vi "Autonomous.vi"() -> ()   [LabVIEW 2018]
doc: "This VI starts when autonomous period begins, and will automatically be terminated when it ends. You can carry out timed or sensor driven operations directly to I/O or to subsystems without needing to return to the caller."
uses:
  Motion_Profiler_Class-master/MotionProfiles.lvclass
  <vilib>/Rock Robotics/WPI/SafetyOutput/WPI_SafetyOutputConfigMenu.ctl
  d1af4e31-2977-4334-b470-f567b7f2c4f2.vi
  <vilib>/Rock Robotics/Network Tables/NT Read String.vi
  <vilib>/Rock Robotics/WPI/Utilities/WPI_GetSetVariantRefNum.vi
  <vilib>/Rock Robotics/Network Tables/NT Read Boolean.vi
panel:
  out "MotionProfiles out":refnum<class "MotionProfiles.lvclass">
  out "Left Motor":T1(graph)
  out "Left Throttle":dbl(graph)
  out "Right Motor":T2(graph)
  out "Right Throttle":dbl(graph)
  out "Right Bottom Buf Count":i32
  out "Left Bottom Buf Count":i32
  out "Right Under Run":bool
  out "Left Under Run":bool
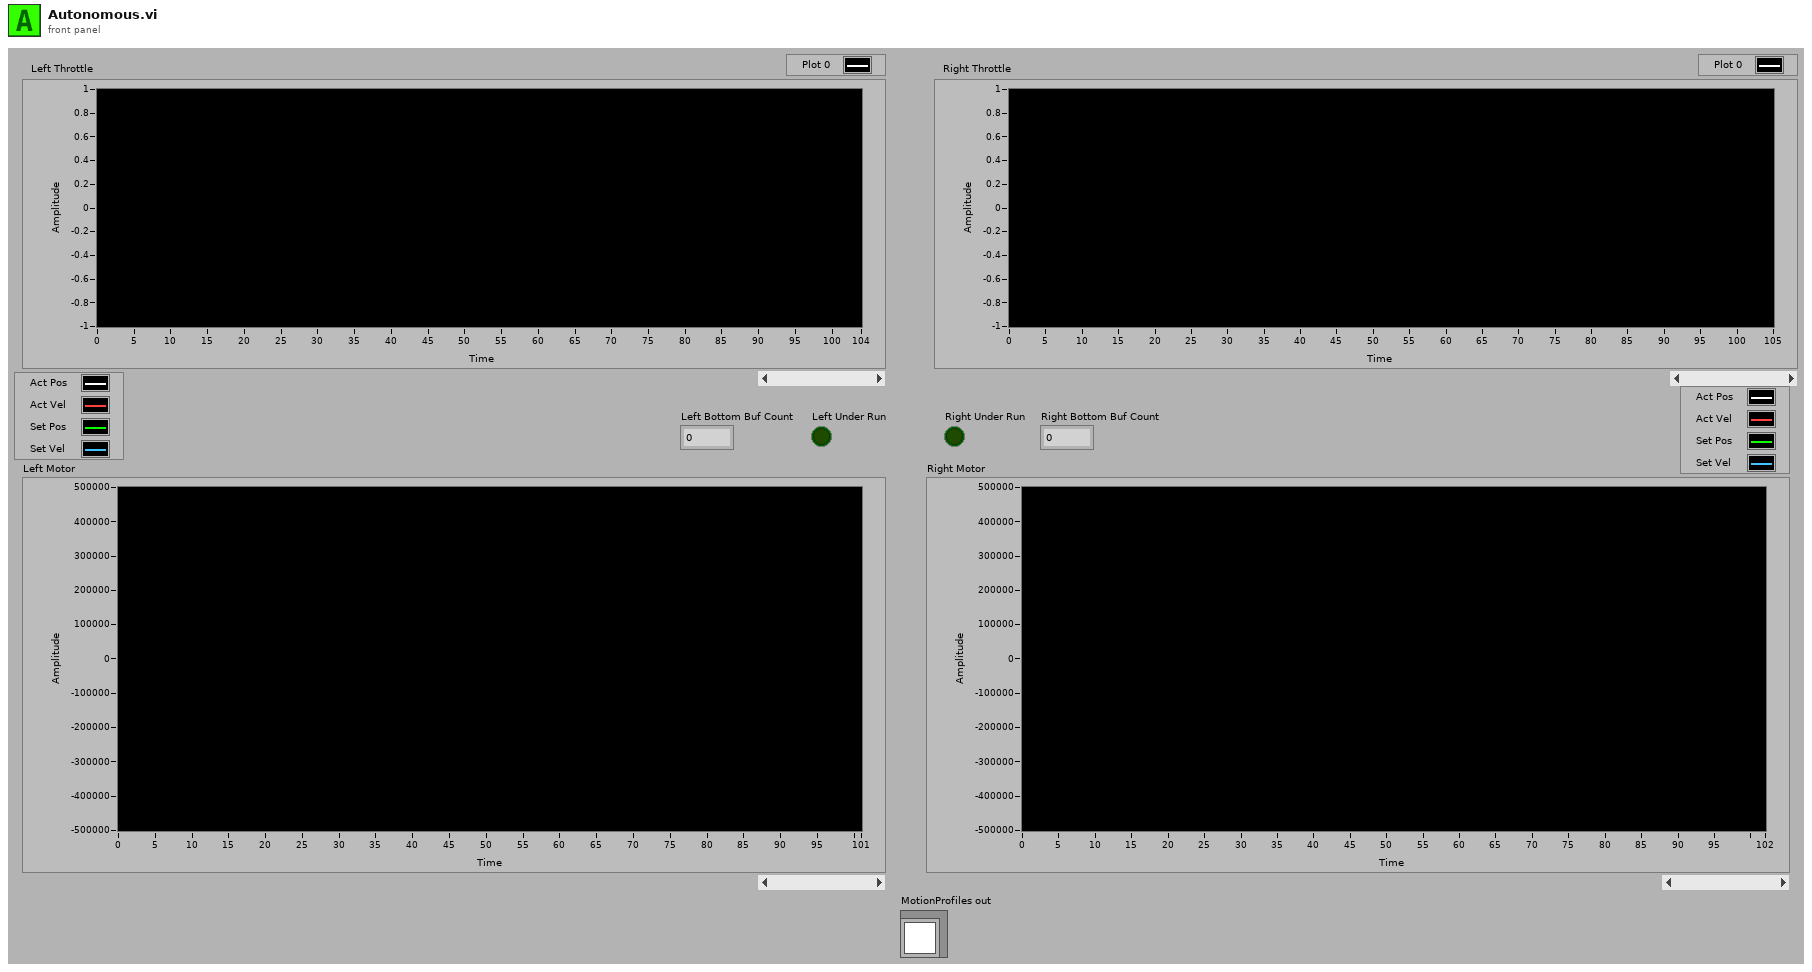
[diagram p1: front panel]
types:
  T1 = cluster{"Set_Pos_(u)":i32, "Set_Pos_(u)":i32, "Act_Vel_(u/100ms)":i32, "Set_Vel_(u/100ms)":i32}
  T2 = cluster{"Set_Vel_(u/100ms)":i32, "Act_Vel_(u/100ms)":i32, "Set_Pos_(u)":i32, "Act_Pos(u)":i32}
  T3 = typedef "WPI_SafetyOutputConfigMenu.ctl" = enum16{"Enable", "Disable"}
  T4 = typedef "WPI_RobotDriveDevRef.ctl" = cluster{"DevStatus":errorcluster, "Motors[]":T5[], "Square Inputs":bool, "Max Output":dbl}
  T5 = typedef "WPI_MotorControlDeviceRef.ctl" = cluster{"DeviceStatus":errorcluster, "Type":T6, "PWM":cluster{"PWM Channel":T7, "DeadBand":T8}, "CAN":cluster{"Device Number":u8, "SetOutput VI Ref":variant, "GetOutput VI Ref":variant, "Enable VI Ref":variant, "Disable VI Ref":variant, "Data":variant}, "Invert":bool, "DIO PWM":cluster{"PWM \"Enable\" Channel":T7, "DIOChannel":T9, "PWM Rate":dbl}}
  T6 = typedef "WPI_MotorControlType.ctl" = enum16{"PWM", "CAN", "DIO PWM"}
  T7 = typedef "FPGA_DIOPWMChannel.ctl" = enum8{"PWM 0", "PWM 1", "PWM 2", "PWM 3", "PWM 4", "PWM 5", "PWM 6", "PWM 7", "PWM 8", "PWM 9", "PWM MXP 0", "PWM MXP 1", "PWM MXP 2", "PWM MXP 3", "PWM MXP 4", "PWM MXP 5", "PWM MXP 6", "PWM MXP 7", "PWM MXP 8", "PWM MXP 9", "Invalid"}
  T8 = typedef "WPI_PWMDeadband.ctl" = cluster{"Name":string, "maxPositivePwm":i32, "minPositivePwm":i32, "centerPwm":i32, "maxNegativePwm":i32, "minNegativePwm":i32, "angularRange":u16}
  T9 = typedef "FPGA_DIOChannel.ctl" = enum8{"DIO 0", "DIO 1", "DIO 2", "DIO 3", "DIO 4", "DIO 5", "DIO 6", "DIO 7", "DIO 8", "DIO 9", "DIO MXP 0", "DIO MXP 1", "DIO MXP 2", "DIO MXP 3", "DIO MXP 4", "DIO MXP 5", "DIO MXP 6", "DIO MXP 7", "DIO MXP 8", "DIO MXP 9", "DIO MXP 10", "DIO MXP 11", "DIO MXP 12", "DIO MXP 13", "DIO MXP 14", "DIO MXP 15", "SPI Port CS1", "SPI Port CS2", "SPI Port CS3", "SPI Port MISO", "SPI Port MOSI", "Invalid"}
  T10 = typedef "MotionProfiles.lvclass/MotionProfile_MP_Class_Status.ctl" = cluster{"Motion Profile Status":cluster{"Top Buffer Remaining":i32, "Top Buffer Count":i32, "Bottom Buffer Count":i32, "Has Underrun?":bool, "Is Underrun?":bool, "Active Point Valid?":bool, "Is Last?":bool, "Profile Slot Select 0":i32, "Output Enable":i32, "Time Duration (ms)":i32, "Profile Slot Select 1":i32}, "TalonState":T11, "MP Is Done":bool, "MP Is Executing":bool, "Set_Vel_(u/100ms)":i32, "Set_Pos_(u)":i32, "Act_Vel_(u/100ms)":i32, "Act_Pos(u)":i32, "Throtle":dbl}
  T11 = typedef "MotionProfiles.lvclass/MotionProfile_TalonSetValueEnum.ctl" = enum16{"Disable", "Enable", "Hold"}
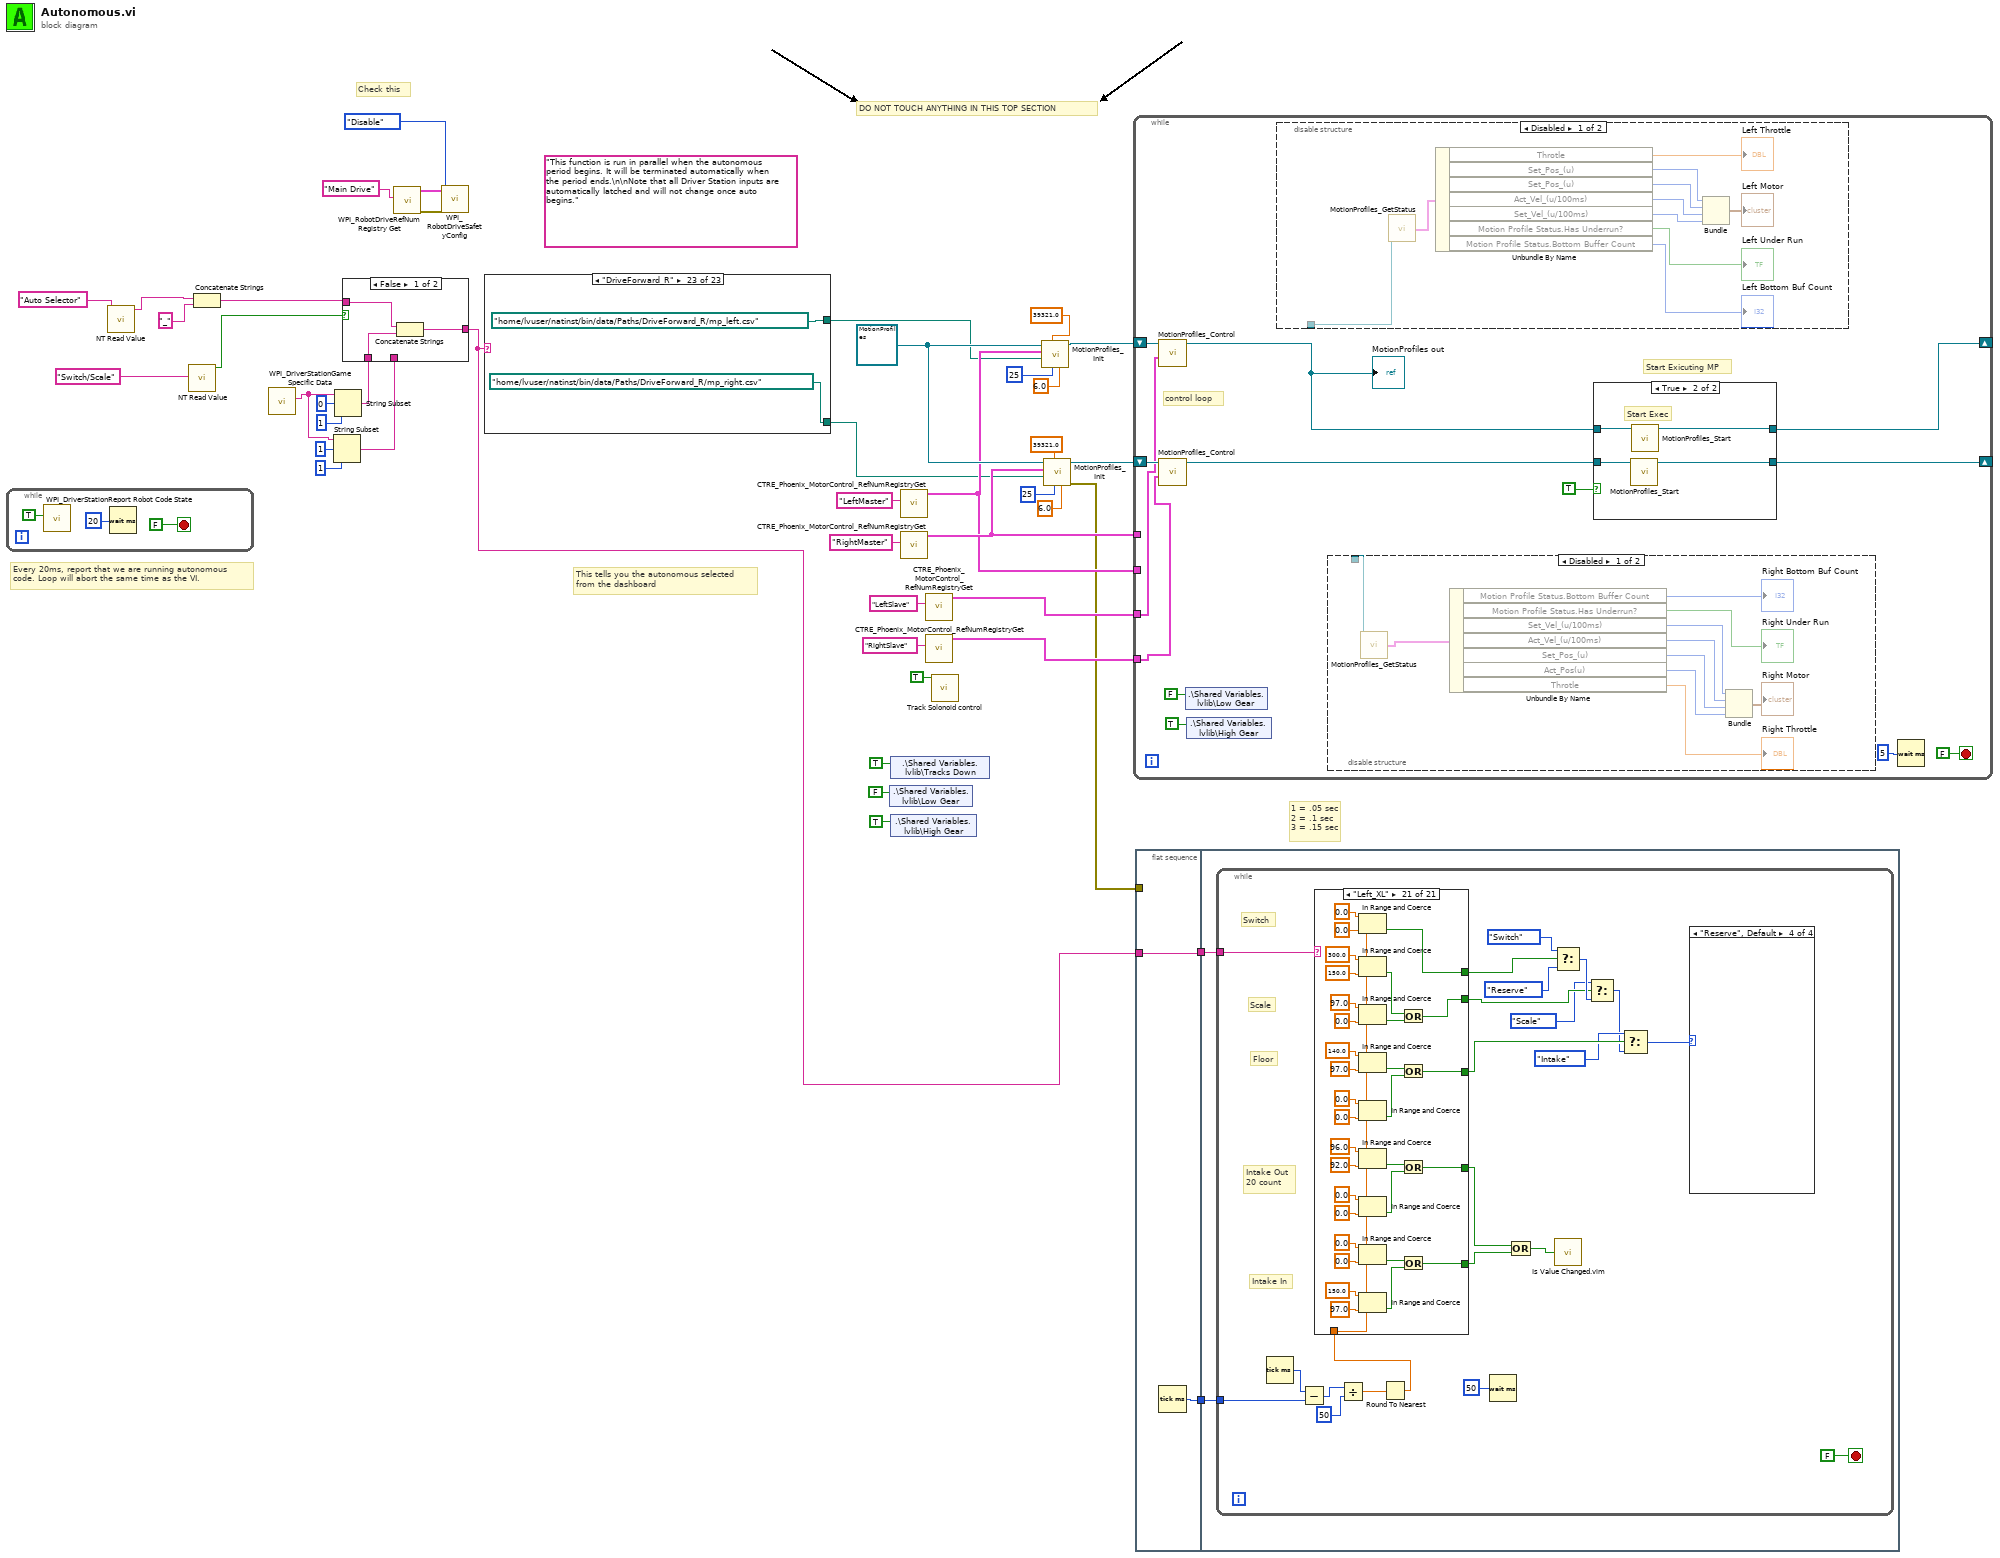
[diagram p0: block diagram]
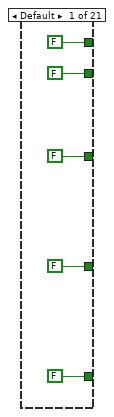
[diagram p5: hidden frame]
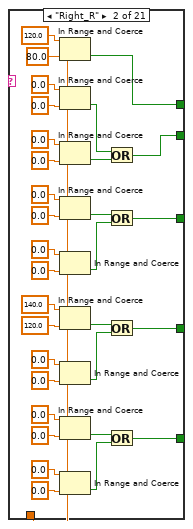
[diagram p6: hidden frame]
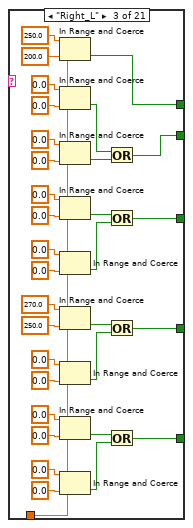
[diagram p7: hidden frame]
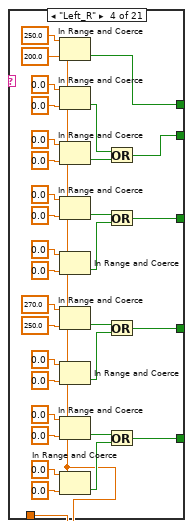
[diagram p8: hidden frame]
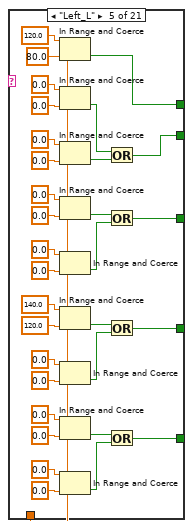
[diagram p9: hidden frame]
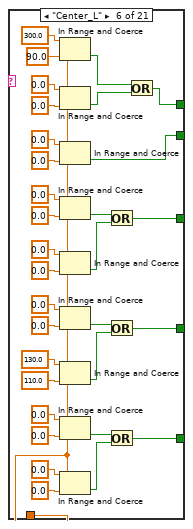
[diagram p10: hidden frame]
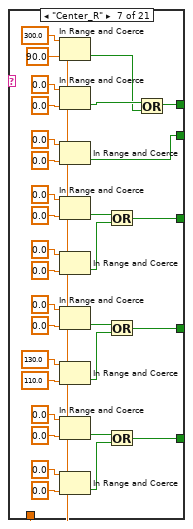
[diagram p11: hidden frame]
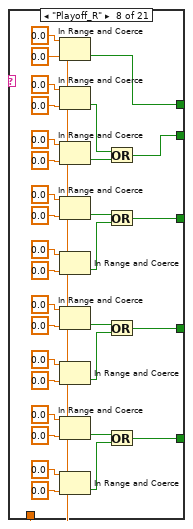
[diagram p12: hidden frame]
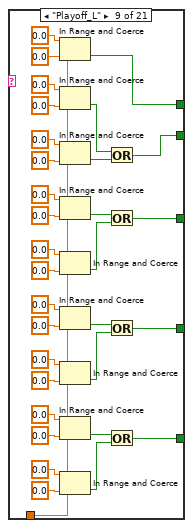
[diagram p13: hidden frame]
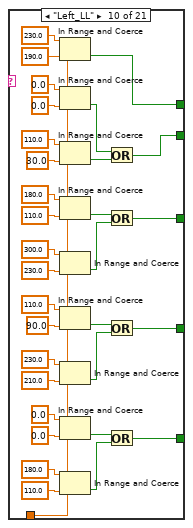
[diagram p14: hidden frame]
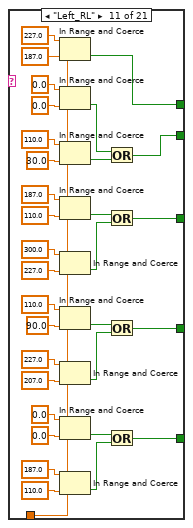
[diagram p15: hidden frame]
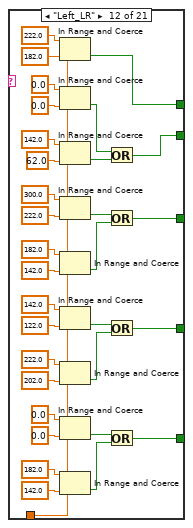
[diagram p16: hidden frame]
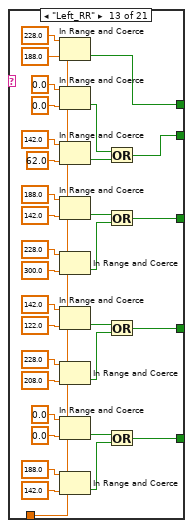
[diagram p17: hidden frame]
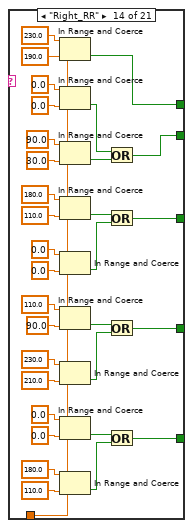
[diagram p18: hidden frame]
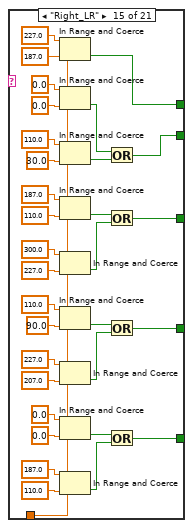
[diagram p19: hidden frame]
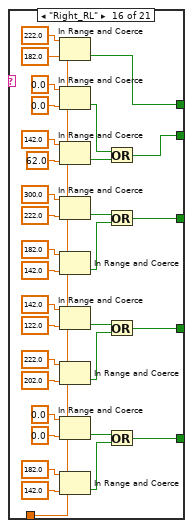
[diagram p20: hidden frame]
diagram:
  w40 = refnum<class "MotionProfiles.lvclass"> refnum ("MotionProfiles.lvclass")
  (unwired) "This function is run in parallel when the autonomous period begins. It will be terminated automatically when the period ends.\n\nNote that all Driver Station inputs are automatically latched and will not change once auto begins."
  # "1 = .05 sec\n2 = .1 sec\n3 = .15 sec"
  # "Check this"
  # "DO NOT TOUCH ANYTHING IN THIS TOP SECTION"
  # "This tells you the autonomous selected\nfrom the dashboard"
  # "Every 20ms, report that we are running autonomous\ncode. Loop will abort the same time as the VI."
  n1 = while {
    stop <- FALSE stop-if-true
    n2 = call <vilib>:"WPI_DriverStationReport Robot Code State.vi"("Autonomous"=TRUE) -> ()  [unwired: 10 in, 1 out]
    n3 = Wait (ms)(milliseconds to wait=u32 20) -> ()  [unwired: 1 out]
  }
  n4 = call-poly <vilib>:"NT Read Value.vi"("Name"="Auto Selector") -> ("String"=w18:string)  [unwired: 9 in, 1 out]
  n5 = call-poly <vilib>:"NT Read Value.vi"("Name"="Switch/Scale") -> ("Boolean"=w4:bool)  [unwired: 9 in, 1 out]
  n6 = Concatenate Strings(w18, "_" ("string")) -> (w8:string)
  n7 = call <vilib>:"WPI_DriverStationGame Specific Data.vi"() -> ("Game Specific Data"=w9:string)  [unwired: 11 in]
  n8 = String Subset(string=w9, offset (0)=1, length (rest)=1 ("length (rest)")) -> (substring=w7:string)
  n9 = String Subset(string=w9, offset (0)=0, length (rest)=1 ("length (rest)")) -> (substring=w6:string)
  n10 = case shown="False" w4 {
    tunnel: w8 -> [w49 w54]
    tunnel: w7 -> [_ w53]
    tunnel: w6 -> [w50 _]
    tunnel: [w48 w52] -> w5
    frame False {
      n11 = Concatenate Strings(w49, w50) -> (w48:string)
    }
    frame True {
      n12 = Concatenate Strings(w54, "X" ("string"), w53) -> (w52:string)
    }
  }
  n13 = call <vilib>:"WPI_RobotDriveRefNum Registry Get.vi"("refnum name"="Main Drive") -> ("error out"=w16:errorcluster, "RobotDriveDevRef"=w15:T4)  [unwired: 9 in]
  n14 = call <vilib>:"WPI_RobotDriveSafetyConfig.vi"("error in (no error)"=w16, "mode"=WPI_SafetyOutputConfigMenu."Disable", "RobotDriveDevRef"=w15) -> ()  [unwired: 7 in, 2 out]
  n15 = case shown="\"DriveForward_R\"" w5 {
    tunnel: [path "" path "/home/lvuser/natinst/bin/data/Paths/Left_L/mp_right.csv" ("file path (use dialog)") path "/home/lvuser/natinst/bin/data/Paths/Left_R/mp_right.csv" ("file path (use dialog)") path "/home/lvuser/natinst/bin/data/Paths/Center_R/mp_right.csv" ("file path (use dialog)") path "/home/lvuser/natinst/bin/data/Paths/Center_L/mp_right.csv" ("file path (use dialog)") path "/home/lvuser/natinst/bin/data/Paths/Right_L/mp_right.csv" ("file path (use dialog)") path "/home/lvuser/natinst/bin/data/Paths/Right_R/mp_right.csv" ("file path (use dialog)") path "/home/lvuser/natinst/bin/data/Paths/Playoff_R/mp_right.csv" ("file path (use dialog)") path "/home/lvuser/natinst/bin/data/Paths/Playoff_L/mp_right.csv" ("file path (use dialog)") path "/home/lvuser/natinst/bin/data/Paths/Left_LL/mp_right.csv" ("file path (use dialog)") path "/home/lvuser/natinst/bin/data/Paths/Left_RL/mp_right.csv" ("file path (use dialog)") path "/home/lvuser/natinst/bin/data/Paths/Left_LR/mp_right.csv" ("file path (use dialog)") path "/home/lvuser/natinst/bin/data/Paths/Left_RR/mp_right.csv" ("file path (use dialog)") path "/home/lvuser/natinst/bin/data/Paths/Right_LL/mp_right.csv" ("file path (use dialog)") path "/home/lvuser/natinst/bin/data/Paths/Right_LR/mp_right.csv" ("file path (use dialog)") path "/home/lvuser/natinst/bin/data/Paths/Right_RL/mp_right.csv" ("file path (use dialog)") path "/home/lvuser/natinst/bin/data/Paths/Right_RR/mp_right.csv" ("file path (use dialog)") path "/home/lvuser/natinst/bin/data/Paths/Left_XL/mp_right.csv" ("file path (use dialog)") path "/home/lvuser/natinst/bin/data/Paths/Left_XR/mp_right.csv" ("file path (use dialog)") path "/home/lvuser/natinst/bin/data/Paths/Right_XR/mp_right.csv" ("file path (use dialog)") path "/home/lvuser/natinst/bin/data/Paths/Right_XL/mp_right.csv" ("file path (use dialog)") path "/home/lvuser/natinst/bin/data/Paths/DriveForward_L/mp_right.csv" ("file path (use dialog)") path "/home/lvuser/natinst/bin/data/Paths/DriveForward_R/mp_right.csv" ("file path (use dialog)")] -> w13
    tunnel: [path "" path "/home/lvuser/natinst/bin/data/Paths/Left_L/mp_left.csv" ("file path (use dialog)") path "/home/lvuser/natinst/bin/data/Paths/Left_R/mp_left.csv" ("file path (use dialog)") path "/home/lvuser/natinst/bin/data/Paths/Center_R/mp_left.csv" ("file path (use dialog)") path "/home/lvuser/natinst/bin/data/Paths/Center_L/mp_left.csv" ("file path (use dialog)") path "/home/lvuser/natinst/bin/data/Paths/Right_L/mp_left.csv" ("file path (use dialog)") path "/home/lvuser/natinst/bin/data/Paths/Right_R/mp_left.csv" ("file path (use dialog)") path "/home/lvuser/natinst/bin/data/Paths/Playoff_R/mp_left.csv" ("file path (use dialog)") path "/home/lvuser/natinst/bin/data/Paths/Playoff_L/mp_left.csv" ("file path (use dialog)") path "/home/lvuser/natinst/bin/data/Paths/Left_LL/mp_left.csv" ("file path (use dialog)") path "/home/lvuser/natinst/bin/data/Paths/Left_RL/mp_left.csv" ("file path (use dialog)") path "/home/lvuser/natinst/bin/data/Paths/Left_LR/mp_left.csv" ("file path (use dialog)") path "/home/lvuser/natinst/bin/data/Paths/Left_RR/mp_left.csv" ("file path (use dialog)") path "/home/lvuser/natinst/bin/data/Paths/Right_LL/mp_left.csv" ("file path (use dialog)") path "/home/lvuser/natinst/bin/data/Paths/Right_LR/mp_left.csv" ("file path (use dialog)") path "/home/lvuser/natinst/bin/data/Paths/Right_RL/mp_left.csv" ("file path (use dialog)") path "/home/lvuser/natinst/bin/data/Paths/Right_RR/mp_left.csv" ("file path (use dialog)") path "/home/lvuser/natinst/bin/data/Paths/Left_XL/mp_left.csv" ("file path (use dialog)") path "/home/lvuser/natinst/bin/data/Paths/Left_XR/mp_left.csv" ("file path (use dialog)") path "/home/lvuser/natinst/bin/data/Paths/Right_XR/mp_left.csv" ("file path (use dialog)") path "/home/lvuser/natinst/bin/data/Paths/Right_XL/mp_left.csv" ("file path (use dialog)") path "/home/lvuser/natinst/bin/data/Paths/DriveForward_L/mp_left.csv" ("file path (use dialog)") path "/home/lvuser/natinst/bin/data/Paths/DriveForward_R/mp_left.csv" ("file path (use dialog)")] -> w12
    frame Default {
    }
    frame "Left_L" {
    }
    frame "Left_R" {
    }
    frame "Center_R" {
    }
    frame "Center_L" {
    }
    frame "Right_L" {
    }
    frame "Right_R" {
    }
    frame "Playoff_R" {
    }
    frame "Playoff_L" {
    }
    frame "Left_LL" {
    }
    frame "Left_RL" {
    }
    frame "Left_LR" {
    }
    frame "Left_RR" {
    }
    frame "Right_LL" {
    }
    frame "Right_LR" {
    }
    frame "Right_RL" {
    }
    frame "Right_RR" {
    }
    frame "Left_XL" {
    }
    frame "Left_XR" {
    }
    frame "Right_XR" {
    }
    frame "Right_XL" {
    }
    frame "DriveForward_L" {
    }
    frame "DriveForward_R" {
    }
  }
  n16 = shared-variable ".\\Shared Variables.lvlib\\Low Gear"(FALSE ("Low Gear")) -> ()  [unwired: 1 in, 1 out]
  n17 = shared-variable ".\\Shared Variables.lvlib\\Tracks Down"(TRUE ("High Gear")) -> ()  [unwired: 1 in, 1 out]
  n18 = shared-variable ".\\Shared Variables.lvlib\\High Gear"(TRUE ("High Gear")) -> ()  [unwired: 1 in, 1 out]
  n19 = call <vilib>:"CTRE_Phoenix_MotorControl_RefNumRegistryGet.vi"("refnum name"="LeftMaster") -> ("PhoenixMotorControlDevRef"=w31:T5)  [unwired: 9 in, 1 out]
  n20 = call <vilib>:"CTRE_Phoenix_MotorControl_RefNumRegistryGet.vi"("refnum name"="RightMaster") -> ("PhoenixMotorControlDevRef"=w32:T5)  [unwired: 9 in, 1 out]
  n21 = call <vilib>:"CTRE_Phoenix_MotorControl_RefNumRegistryGet.vi"("refnum name"="LeftSlave") -> ("PhoenixMotorControlDevRef"=w25:T5)  [unwired: 9 in, 1 out]
  n22 = call <vilib>:"CTRE_Phoenix_MotorControl_RefNumRegistryGet.vi"("refnum name"="RightSlave") -> ("PhoenixMotorControlDevRef"=w24:T5)  [unwired: 9 in, 1 out]
  n23 = call "Track Solonoid control.vi"("Manual Tracks"=TRUE) -> ()  [unwired: 11 in]
  n24 = call "MotionProfiles_Init.vi"("Wheel_Diameter (in)"=6.0 ("Wheel Diameter"), "MP_Frame_Rate_(ms)"=25, "Encoder_CPR_4x"=39321.0, "CSV File Path"=w12, "PhoenixMotorControlDevRef"=w31, "MotionProfiles in"=w40) -> ("MotionProfiles out"=w43:refnum<class "MotionProfiles.lvclass">)  [unwired: 4 in, 1 out]
  n25 = call "MotionProfiles_Init.vi"("Wheel_Diameter (in)"=6.0, "MP_Frame_Rate_(ms)"=25, "Encoder_CPR_4x"=39321.0, "CSV File Path"=w13, "PhoenixMotorControlDevRef"=w32, "MotionProfiles in"=w40) -> ("error out"=w23:errorcluster, "MotionProfiles out"=w41:refnum<class "MotionProfiles.lvclass">)  [unwired: 4 in]
  n26 = while {
    shift-right: [w108] -> _
    shift-left: w43 -> [w111]
    shift-right: [w109] -> _
    shift-left: w41 -> [w110]
    tunnel: w32 -> [_]
    tunnel: w31 -> [_]
    tunnel: w25 -> [w106]
    tunnel: w24 -> [w105]
    stop <- FALSE stop-if-true
    # "control loop"
    # "Start Exicuting MP"
    n27 = call "MotionProfiles_Control.vi"("PhoenixMotorControlDevRef Slave"=w106, "MotionProfiles in"=w111) -> ("MotionProfiles out"=w101:refnum<class "MotionProfiles.lvclass">)  [unwired: 8 in, 1 out]
    "MotionProfiles out" <- w101
    n28 = call "MotionProfiles_Control.vi"("PhoenixMotorControlDevRef Slave"=w105, "MotionProfiles in"=w110) -> ("MotionProfiles out"=w102:refnum<class "MotionProfiles.lvclass">)  [unwired: 8 in, 1 out]
    n29 = shared-variable ".\\Shared Variables.lvlib\\Low Gear"(FALSE ("Low Gear")) -> ()  [unwired: 1 in, 1 out]
    n30 = shared-variable ".\\Shared Variables.lvlib\\High Gear"(TRUE ("High Gear")) -> ()  [unwired: 1 in, 1 out]
    n31 = disable-structure shown="Disabled" {
      disable-tunnel: _ -> [w133 _]
      frame Disabled {
        n32 = call "MotionProfiles_GetStatus.vi"("MotionProfiles in"=w133) -> ("MP_Class_Status"=w132:T10)  [unwired: 12 in, 2 out]
        n33 = Unbundle By Name(w132) -> ("Throtle"=→"Left Throttle":dbl, "Set_Pos_(u)"=w125:i32, "Set_Pos_(u)"=w126:i32, "Act_Vel_(u/100ms)"=w127:i32, "Set_Vel_(u/100ms)"=w128:i32, "Motion Profile Status.Has Underrun?"=→"Left Under Run":bool, "Motion Profile Status.Bottom Buffer Count"=→"Left Bottom Buf Count":i32)
        n34 = Bundle("Set_Pos_(u)"=w125, "Set_Pos_(u)"=w126, "Act_Vel_(u/100ms)"=w127, "Set_Vel_(u/100ms)"=w128) -> (→"Left Motor":T1)  [unwired: 1 in]
      }
      frame Enabled {
      }
    }
    n35 = disable-structure shown="Disabled" {
      disable-tunnel: _ -> [w123 _]
      frame Disabled {
        n36 = call "MotionProfiles_GetStatus.vi"("MotionProfiles in"=w123) -> ("MP_Class_Status"=w122:T10)  [unwired: 12 in, 2 out]
        n37 = Unbundle By Name(w122) -> ("Motion Profile Status.Bottom Buffer Count"=→"Right Bottom Buf Count":i32, "Motion Profile Status.Has Underrun?"=→"Right Under Run":bool, "Set_Vel_(u/100ms)"=w118:i32, "Act_Vel_(u/100ms)"=w117:i32, "Set_Pos_(u)"=w116:i32, "Act_Pos(u)"=w115:i32, "Throtle"=→"Right Throttle":dbl)
        n38 = Bundle("Set_Vel_(u/100ms)"=w118, "Act_Vel_(u/100ms)"=w117, "Set_Pos_(u)"=w116, "Act_Pos(u)"=w115) -> (→"Right Motor":T2)  [unwired: 1 in]
      }
      frame Enabled {
      }
    }
    n39 = case shown="True" TRUE {
      tunnel: w101 -> [w135 w139]
      tunnel: w102 -> [w134 w137]
      tunnel: [w134 w136] -> w109
      tunnel: [w135 w138] -> w108
      frame False {
      }
      frame True {
        # "Start Exec"
        n40 = call "MotionProfiles_Start.vi"("MotionProfiles in"=w137) -> ("MotionProfiles out"=w136:refnum<class "MotionProfiles.lvclass">)  [unwired: 9 in, 1 out]
        n41 = call "MotionProfiles_Start.vi"("MotionProfiles in"=w139) -> ("MotionProfiles out"=w138:refnum<class "MotionProfiles.lvclass">)  [unwired: 9 in, 1 out]
      }
    }
    n42 = Wait (ms)(milliseconds to wait=u32 5) -> ()  [unwired: 1 out]
  }
  n43 = flat-sequence {
    tunnel: [w141] -> w2
    tunnel: [w140] -> w1
    tunnel: w5 -> [w140]
    tunnel: w23 -> [_]
    tunnel: w2 -> [w143]
    tunnel: w1 -> [w142]
    frame #0 {
      n44 = Tick Count (ms)() -> (millisecond timer value=w141:u32)
    }
    frame #1 {
      n45 = while {
        tunnel: w142 -> [w161]
        tunnel: w143 -> [w162]
        stop <- FALSE stop-if-true
        # "Intake In"
        # "Intake Out\n20 count"
        # "Floor"
        # "Scale"
        # "Switch"
        n46 = Tick Count (ms)() -> (millisecond timer value=w164:u32)
        n47 = Subtract(x=w164, y=w162) -> (x-y=w156:u32)
        n48 = Divide(x=w156, y=u32 50) -> (x/y=w163:dbl)
        n49 = Round To Nearest(number=w163) -> (nearest integer value=w160:dbl)
        n50 = case shown="\"Left_XL\"" w161 {
          tunnel: w160 -> [_ w171 w203 w235 w267 w303 w334 w363 w395 w427 w459 w491 w523 w555 w587 w619 w651 w683 w715 w747 w779]
          tunnel: [FALSE w202 w234 w266 w298 w302 w332 w394 w426 w458 w490 w522 w554 w586 w618 w650 w682 w714 w746 w778 w810] -> w152
          tunnel: [FALSE w199 w231 w263 w295 w328 w360 w391 w423 w455 w487 w519 w551 w583 w615 w647 w679 w711 w743 w775 w807] -> w145
          tunnel: [FALSE w196 w228 w260 w292 w325 w357 w388 w420 w452 w484 w516 w548 w580 w612 w644 w676 w708 w740 w772 w804] -> w157
          tunnel: [FALSE w173 w205 w237 w269 w304 w335 w365 w397 w429 w461 w493 w525 w557 w589 w621 w653 w685 w717 w749 w781] -> w149
          tunnel: [FALSE w172 w204 w236 w268 w299 w331 w364 w396 w428 w460 w492 w524 w556 w588 w620 w652 w684 w716 w748 w780] -> w150
          frame Default {
          }
          frame "Right_R" {
            n51 = In Range and Coerce(upper limit=120.0, x=w171, lower limit=80.0) -> (In Range?=w202:bool)  [unwired: 1 out]
            n52 = In Range and Coerce(upper limit=0.0, x=w171, lower limit=0.0) -> (In Range?=w185:bool)  [unwired: 1 out]
            n53 = In Range and Coerce(upper limit=0.0, x=w171, lower limit=0.0) -> (In Range?=w184:bool)  [unwired: 1 out]
            n54 = In Range and Coerce(upper limit=0.0, x=w171, lower limit=0.0) -> (In Range?=w179:bool)  [unwired: 1 out]
            n55 = In Range and Coerce(upper limit=0.0, x=w171, lower limit=0.0) -> (In Range?=w178:bool)  [unwired: 1 out]
            n56 = In Range and Coerce(upper limit=140.0, x=w171, lower limit=120.0) -> (In Range?=w198:bool)  [unwired: 1 out]
            n57 = In Range and Coerce(upper limit=0.0 ("x"), x=w171, lower limit=0.0) -> (In Range?=w197:bool)  [unwired: 1 out]
            n58 = In Range and Coerce(upper limit=0.0, x=w171, lower limit=0.0) -> (In Range?=w201:bool)  [unwired: 1 out]
            n59 = In Range and Coerce(upper limit=0.0, x=w171, lower limit=0.0) -> (In Range?=w200:bool)  [unwired: 1 out]
            n60 = Or(x=w185, y=w184) -> (x .or. y?=w172:bool)
            n61 = Or(x=w179, y=w178) -> (x .or. y?=w173:bool)
            n62 = Or(x=w198, y=w197) -> (x .or. y?=w196:bool)
            n63 = Or(x=w201, y=w200) -> (x .or. y?=w199:bool)
          }
          frame "Right_L" {
            n64 = In Range and Coerce(upper limit=250.0, x=w203, lower limit=200.0) -> (In Range?=w234:bool)  [unwired: 1 out]
            n65 = In Range and Coerce(upper limit=0.0, x=w203, lower limit=0.0) -> (In Range?=w217:bool)  [unwired: 1 out]
            n66 = In Range and Coerce(upper limit=0.0, x=w203, lower limit=0.0) -> (In Range?=w216:bool)  [unwired: 1 out]
            n67 = In Range and Coerce(upper limit=0.0, x=w203, lower limit=0.0) -> (In Range?=w211:bool)  [unwired: 1 out]
            n68 = In Range and Coerce(upper limit=0.0, x=w203, lower limit=0.0) -> (In Range?=w210:bool)  [unwired: 1 out]
            n69 = In Range and Coerce(upper limit=270.0, x=w203, lower limit=250.0) -> (In Range?=w230:bool)  [unwired: 1 out]
            n70 = In Range and Coerce(upper limit=0.0 ("x"), x=w203, lower limit=0.0) -> (In Range?=w229:bool)  [unwired: 1 out]
            n71 = In Range and Coerce(upper limit=0.0, x=w203, lower limit=0.0) -> (In Range?=w233:bool)  [unwired: 1 out]
            n72 = In Range and Coerce(upper limit=0.0, x=w203, lower limit=0.0) -> (In Range?=w232:bool)  [unwired: 1 out]
            n73 = Or(x=w217, y=w216) -> (x .or. y?=w204:bool)
            n74 = Or(x=w211, y=w210) -> (x .or. y?=w205:bool)
            n75 = Or(x=w230, y=w229) -> (x .or. y?=w228:bool)
            n76 = Or(x=w233, y=w232) -> (x .or. y?=w231:bool)
          }
          frame "Left_R" {
            n77 = In Range and Coerce(upper limit=250.0, x=w235, lower limit=200.0) -> (In Range?=w266:bool)  [unwired: 1 out]
            n78 = In Range and Coerce(upper limit=0.0, x=w235, lower limit=0.0) -> (In Range?=w249:bool)  [unwired: 1 out]
            n79 = In Range and Coerce(upper limit=0.0, x=w235, lower limit=0.0) -> (In Range?=w248:bool)  [unwired: 1 out]
            n80 = In Range and Coerce(upper limit=0.0, x=w235, lower limit=0.0) -> (In Range?=w243:bool)  [unwired: 1 out]
            n81 = In Range and Coerce(upper limit=0.0, x=w235, lower limit=0.0) -> (In Range?=w242:bool)  [unwired: 1 out]
            n82 = In Range and Coerce(upper limit=270.0, x=w235, lower limit=250.0) -> (In Range?=w262:bool)  [unwired: 1 out]
            n83 = In Range and Coerce(upper limit=0.0 ("x"), x=w235, lower limit=0.0) -> (In Range?=w261:bool)  [unwired: 1 out]
            n84 = In Range and Coerce(upper limit=0.0, x=w235, lower limit=0.0) -> (In Range?=w265:bool)  [unwired: 1 out]
            n85 = In Range and Coerce(upper limit=0.0, x=w235, lower limit=0.0) -> (In Range?=w264:bool)  [unwired: 1 out]
            n86 = Or(x=w249, y=w248) -> (x .or. y?=w236:bool)
            n87 = Or(x=w243, y=w242) -> (x .or. y?=w237:bool)
            n88 = Or(x=w262, y=w261) -> (x .or. y?=w260:bool)
            n89 = Or(x=w265, y=w264) -> (x .or. y?=w263:bool)
          }
          frame "Left_L" {
            n90 = In Range and Coerce(upper limit=120.0, x=w267, lower limit=80.0) -> (In Range?=w298:bool)  [unwired: 1 out]
            n91 = In Range and Coerce(upper limit=0.0, x=w267, lower limit=0.0) -> (In Range?=w281:bool)  [unwired: 1 out]
            n92 = In Range and Coerce(upper limit=0.0, x=w267, lower limit=0.0) -> (In Range?=w280:bool)  [unwired: 1 out]
            n93 = In Range and Coerce(upper limit=0.0, x=w267, lower limit=0.0) -> (In Range?=w275:bool)  [unwired: 1 out]
            n94 = In Range and Coerce(upper limit=0.0, x=w267, lower limit=0.0) -> (In Range?=w274:bool)  [unwired: 1 out]
            n95 = In Range and Coerce(upper limit=140.0, x=w267, lower limit=120.0) -> (In Range?=w294:bool)  [unwired: 1 out]
            n96 = In Range and Coerce(upper limit=0.0 ("x"), x=w267, lower limit=0.0) -> (In Range?=w293:bool)  [unwired: 1 out]
            n97 = In Range and Coerce(upper limit=0.0, x=w267, lower limit=0.0) -> (In Range?=w297:bool)  [unwired: 1 out]
            n98 = In Range and Coerce(upper limit=0.0, x=w267, lower limit=0.0) -> (In Range?=w296:bool)  [unwired: 1 out]
            n99 = Or(x=w281, y=w280) -> (x .or. y?=w268:bool)
            n100 = Or(x=w275, y=w274) -> (x .or. y?=w269:bool)
            n101 = Or(x=w294, y=w293) -> (x .or. y?=w292:bool)
            n102 = Or(x=w297, y=w296) -> (x .or. y?=w295:bool)
          }
          frame "Center_L" {
            n103 = In Range and Coerce(upper limit=300.0, x=w303, lower limit=90.0) -> (In Range?=w301:bool)  [unwired: 1 out]
            n104 = In Range and Coerce(upper limit=0.0, x=w303, lower limit=0.0) -> (In Range?=w300:bool)  [unwired: 1 out]
            n105 = In Range and Coerce(upper limit=0.0, x=w303, lower limit=0.0) -> (In Range?=w299:bool)  [unwired: 1 out]
            n106 = In Range and Coerce(upper limit=0.0, x=w303, lower limit=0.0) -> (In Range?=w310:bool)  [unwired: 1 out]
            n107 = In Range and Coerce(upper limit=0.0, x=w303, lower limit=0.0) -> (In Range?=w309:bool)  [unwired: 1 out]
            n108 = In Range and Coerce(upper limit=0.0, x=w303, lower limit=0.0) -> (In Range?=w327:bool)  [unwired: 1 out]
            n109 = In Range and Coerce(upper limit=130.0 ("x"), x=w303, lower limit=110.0) -> (In Range?=w326:bool)  [unwired: 1 out]
            n110 = In Range and Coerce(upper limit=0.0, x=w303, lower limit=0.0) -> (In Range?=w330:bool)  [unwired: 1 out]
            n111 = In Range and Coerce(upper limit=0.0, x=w303, lower limit=0.0) -> (In Range?=w329:bool)  [unwired: 1 out]
            n112 = Or(x=w310, y=w309) -> (x .or. y?=w304:bool)
            n113 = Or(x=w327, y=w326) -> (x .or. y?=w325:bool)
            n114 = Or(x=w330, y=w329) -> (x .or. y?=w328:bool)
            n115 = Or(x=w301, y=w300) -> (x .or. y?=w302:bool)
          }
          frame "Center_R" {
            n116 = In Range and Coerce(upper limit=300.0, x=w334, lower limit=90.0) -> (In Range?=w333:bool)  [unwired: 1 out]
            n117 = In Range and Coerce(upper limit=0.0, x=w334, lower limit=0.0) -> (In Range?=w346:bool)  [unwired: 1 out]
            n118 = In Range and Coerce(upper limit=0.0, x=w334, lower limit=0.0) -> (In Range?=w331:bool)  [unwired: 1 out]
            n119 = In Range and Coerce(upper limit=0.0, x=w334, lower limit=0.0) -> (In Range?=w341:bool)  [unwired: 1 out]
            n120 = In Range and Coerce(upper limit=0.0, x=w334, lower limit=0.0) -> (In Range?=w340:bool)  [unwired: 1 out]
            n121 = In Range and Coerce(upper limit=0.0, x=w334, lower limit=0.0) -> (In Range?=w359:bool)  [unwired: 1 out]
            n122 = In Range and Coerce(upper limit=130.0 ("x"), x=w334, lower limit=110.0) -> (In Range?=w358:bool)  [unwired: 1 out]
            n123 = In Range and Coerce(upper limit=0.0, x=w334, lower limit=0.0) -> (In Range?=w362:bool)  [unwired: 1 out]
            n124 = In Range and Coerce(upper limit=0.0, x=w334, lower limit=0.0) -> (In Range?=w361:bool)  [unwired: 1 out]
            n125 = Or(x=w341, y=w340) -> (x .or. y?=w335:bool)
            n126 = Or(x=w359, y=w358) -> (x .or. y?=w357:bool)
            n127 = Or(x=w362, y=w361) -> (x .or. y?=w360:bool)
            n128 = Or(x=w346, y=w333) -> (x .or. y?=w332:bool)
          }
          frame "Playoff_R" {
            n129 = In Range and Coerce(upper limit=0.0, x=w363, lower limit=0.0) -> (In Range?=w394:bool)  [unwired: 1 out]
            n130 = In Range and Coerce(upper limit=0.0, x=w363, lower limit=0.0) -> (In Range?=w377:bool)  [unwired: 1 out]
            n131 = In Range and Coerce(upper limit=0.0, x=w363, lower limit=0.0) -> (In Range?=w376:bool)  [unwired: 1 out]
            n132 = In Range and Coerce(upper limit=0.0, x=w363, lower limit=0.0) -> (In Range?=w371:bool)  [unwired: 1 out]
            n133 = In Range and Coerce(upper limit=0.0, x=w363, lower limit=0.0) -> (In Range?=w370:bool)  [unwired: 1 out]
            n134 = In Range and Coerce(upper limit=0.0, x=w363, lower limit=0.0) -> (In Range?=w390:bool)  [unwired: 1 out]
            n135 = In Range and Coerce(upper limit=0.0 ("x"), x=w363, lower limit=0.0) -> (In Range?=w389:bool)  [unwired: 1 out]
            n136 = In Range and Coerce(upper limit=0.0, x=w363, lower limit=0.0) -> (In Range?=w393:bool)  [unwired: 1 out]
            n137 = In Range and Coerce(upper limit=0.0, x=w363, lower limit=0.0) -> (In Range?=w392:bool)  [unwired: 1 out]
            n138 = Or(x=w377, y=w376) -> (x .or. y?=w364:bool)
            n139 = Or(x=w371, y=w370) -> (x .or. y?=w365:bool)
            n140 = Or(x=w390, y=w389) -> (x .or. y?=w388:bool)
            n141 = Or(x=w393, y=w392) -> (x .or. y?=w391:bool)
          }
          frame "Playoff_L" {
            n142 = In Range and Coerce(upper limit=0.0, x=w395, lower limit=0.0) -> (In Range?=w426:bool)  [unwired: 1 out]
            n143 = In Range and Coerce(upper limit=0.0, x=w395, lower limit=0.0) -> (In Range?=w409:bool)  [unwired: 1 out]
            n144 = In Range and Coerce(upper limit=0.0, x=w395, lower limit=0.0) -> (In Range?=w408:bool)  [unwired: 1 out]
            n145 = In Range and Coerce(upper limit=0.0, x=w395, lower limit=0.0) -> (In Range?=w403:bool)  [unwired: 1 out]
            n146 = In Range and Coerce(upper limit=0.0, x=w395, lower limit=0.0) -> (In Range?=w402:bool)  [unwired: 1 out]
            n147 = In Range and Coerce(upper limit=0.0, x=w395, lower limit=0.0) -> (In Range?=w422:bool)  [unwired: 1 out]
            n148 = In Range and Coerce(upper limit=0.0 ("x"), x=w395, lower limit=0.0) -> (In Range?=w421:bool)  [unwired: 1 out]
            n149 = In Range and Coerce(upper limit=0.0, x=w395, lower limit=0.0) -> (In Range?=w425:bool)  [unwired: 1 out]
            n150 = In Range and Coerce(upper limit=0.0, x=w395, lower limit=0.0) -> (In Range?=w424:bool)  [unwired: 1 out]
            n151 = Or(x=w409, y=w408) -> (x .or. y?=w396:bool)
            n152 = Or(x=w403, y=w402) -> (x .or. y?=w397:bool)
            n153 = Or(x=w422, y=w421) -> (x .or. y?=w420:bool)
            n154 = Or(x=w425, y=w424) -> (x .or. y?=w423:bool)
          }
          frame "Left_LL" {
            n155 = In Range and Coerce(upper limit=230.0, x=w427, lower limit=190.0) -> (In Range?=w458:bool)  [unwired: 1 out]
            n156 = In Range and Coerce(upper limit=0.0, x=w427, lower limit=0.0) -> (In Range?=w441:bool)  [unwired: 1 out]
            n157 = In Range and Coerce(upper limit=110.0, x=w427, lower limit=30.0) -> (In Range?=w440:bool)  [unwired: 1 out]
            n158 = In Range and Coerce(upper limit=180.0, x=w427, lower limit=110.0) -> (In Range?=w435:bool)  [unwired: 1 out]
            n159 = In Range and Coerce(upper limit=300.0, x=w427, lower limit=230.0) -> (In Range?=w434:bool)  [unwired: 1 out]
            n160 = In Range and Coerce(upper limit=110.0, x=w427, lower limit=90.0) -> (In Range?=w454:bool)  [unwired: 1 out]
            n161 = In Range and Coerce(upper limit=230.0 ("x"), x=w427, lower limit=210.0) -> (In Range?=w453:bool)  [unwired: 1 out]
            n162 = In Range and Coerce(upper limit=0.0, x=w427, lower limit=0.0) -> (In Range?=w457:bool)  [unwired: 1 out]
            n163 = In Range and Coerce(upper limit=180.0, x=w427, lower limit=110.0) -> (In Range?=w456:bool)  [unwired: 1 out]
            n164 = Or(x=w441, y=w440) -> (x .or. y?=w428:bool)
            n165 = Or(x=w435, y=w434) -> (x .or. y?=w429:bool)
            n166 = Or(x=w454, y=w453) -> (x .or. y?=w452:bool)
            n167 = Or(x=w457, y=w456) -> (x .or. y?=w455:bool)
          }
          frame "Left_RL" {
            n168 = In Range and Coerce(upper limit=227.0, x=w459, lower limit=187.0) -> (In Range?=w490:bool)  [unwired: 1 out]
            n169 = In Range and Coerce(upper limit=0.0, x=w459, lower limit=0.0) -> (In Range?=w473:bool)  [unwired: 1 out]
            n170 = In Range and Coerce(upper limit=110.0, x=w459, lower limit=30.0) -> (In Range?=w472:bool)  [unwired: 1 out]
            n171 = In Range and Coerce(upper limit=187.0, x=w459, lower limit=110.0) -> (In Range?=w467:bool)  [unwired: 1 out]
            n172 = In Range and Coerce(upper limit=300.0, x=w459, lower limit=227.0) -> (In Range?=w466:bool)  [unwired: 1 out]
            n173 = In Range and Coerce(upper limit=110.0, x=w459, lower limit=90.0) -> (In Range?=w486:bool)  [unwired: 1 out]
            n174 = In Range and Coerce(upper limit=227.0 ("x"), x=w459, lower limit=207.0) -> (In Range?=w485:bool)  [unwired: 1 out]
            n175 = In Range and Coerce(upper limit=0.0, x=w459, lower limit=0.0) -> (In Range?=w489:bool)  [unwired: 1 out]
            n176 = In Range and Coerce(upper limit=187.0, x=w459, lower limit=110.0) -> (In Range?=w488:bool)  [unwired: 1 out]
            n177 = Or(x=w473, y=w472) -> (x .or. y?=w460:bool)
            n178 = Or(x=w467, y=w466) -> (x .or. y?=w461:bool)
            n179 = Or(x=w486, y=w485) -> (x .or. y?=w484:bool)
            n180 = Or(x=w489, y=w488) -> (x .or. y?=w487:bool)
          }
          frame "Left_LR" {
            n181 = In Range and Coerce(upper limit=222.0, x=w491, lower limit=182.0) -> (In Range?=w522:bool)  [unwired: 1 out]
            n182 = In Range and Coerce(upper limit=0.0, x=w491, lower limit=0.0) -> (In Range?=w505:bool)  [unwired: 1 out]
            n183 = In Range and Coerce(upper limit=142.0, x=w491, lower limit=62.0) -> (In Range?=w504:bool)  [unwired: 1 out]
            n184 = In Range and Coerce(upper limit=300.0, x=w491, lower limit=222.0) -> (In Range?=w499:bool)  [unwired: 1 out]
            n185 = In Range and Coerce(upper limit=182.0, x=w491, lower limit=142.0) -> (In Range?=w498:bool)  [unwired: 1 out]
            n186 = In Range and Coerce(upper limit=142.0, x=w491, lower limit=122.0) -> (In Range?=w518:bool)  [unwired: 1 out]
            n187 = In Range and Coerce(upper limit=222.0 ("x"), x=w491, lower limit=202.0) -> (In Range?=w517:bool)  [unwired: 1 out]
            n188 = In Range and Coerce(upper limit=0.0, x=w491, lower limit=0.0) -> (In Range?=w521:bool)  [unwired: 1 out]
            n189 = In Range and Coerce(upper limit=182.0, x=w491, lower limit=142.0) -> (In Range?=w520:bool)  [unwired: 1 out]
            n190 = Or(x=w505, y=w504) -> (x .or. y?=w492:bool)
            n191 = Or(x=w499, y=w498) -> (x .or. y?=w493:bool)
            n192 = Or(x=w518, y=w517) -> (x .or. y?=w516:bool)
            n193 = Or(x=w521, y=w520) -> (x .or. y?=w519:bool)
          }
          frame "Left_RR" {
            n194 = In Range and Coerce(upper limit=228.0, x=w523, lower limit=188.0) -> (In Range?=w554:bool)  [unwired: 1 out]
            n195 = In Range and Coerce(upper limit=0.0, x=w523, lower limit=0.0) -> (In Range?=w537:bool)  [unwired: 1 out]
            n196 = In Range and Coerce(upper limit=142.0, x=w523, lower limit=62.0) -> (In Range?=w536:bool)  [unwired: 1 out]
            n197 = In Range and Coerce(upper limit=188.0, x=w523, lower limit=142.0) -> (In Range?=w531:bool)  [unwired: 1 out]
            n198 = In Range and Coerce(upper limit=228.0, x=w523, lower limit=300.0) -> (In Range?=w530:bool)  [unwired: 1 out]
            n199 = In Range and Coerce(upper limit=142.0, x=w523, lower limit=122.0) -> (In Range?=w550:bool)  [unwired: 1 out]
            n200 = In Range and Coerce(upper limit=228.0 ("x"), x=w523, lower limit=208.0) -> (In Range?=w549:bool)  [unwired: 1 out]
            n201 = In Range and Coerce(upper limit=0.0, x=w523, lower limit=0.0) -> (In Range?=w553:bool)  [unwired: 1 out]
            n202 = In Range and Coerce(upper limit=188.0, x=w523, lower limit=142.0) -> (In Range?=w552:bool)  [unwired: 1 out]
            n203 = Or(x=w537, y=w536) -> (x .or. y?=w524:bool)
            n204 = Or(x=w531, y=w530) -> (x .or. y?=w525:bool)
            n205 = Or(x=w550, y=w549) -> (x .or. y?=w548:bool)
            n206 = Or(x=w553, y=w552) -> (x .or. y?=w551:bool)
          }
          frame "Right_RR" {
            n207 = In Range and Coerce(upper limit=230.0, x=w555, lower limit=190.0) -> (In Range?=w586:bool)  [unwired: 1 out]
            n208 = In Range and Coerce(upper limit=0.0, x=w555, lower limit=0.0) -> (In Range?=w569:bool)  [unwired: 1 out]
            n209 = In Range and Coerce(upper limit=90.0, x=w555, lower limit=30.0) -> (In Range?=w568:bool)  [unwired: 1 out]
            n210 = In Range and Coerce(upper limit=180.0, x=w555, lower limit=110.0) -> (In Range?=w563:bool)  [unwired: 1 out]
            n211 = In Range and Coerce(upper limit=0.0, x=w555, lower limit=0.0) -> (In Range?=w562:bool)  [unwired: 1 out]
            n212 = In Range and Coerce(upper limit=110.0, x=w555, lower limit=90.0) -> (In Range?=w582:bool)  [unwired: 1 out]
            n213 = In Range and Coerce(upper limit=230.0 ("x"), x=w555, lower limit=210.0) -> (In Range?=w581:bool)  [unwired: 1 out]
            n214 = In Range and Coerce(upper limit=0.0, x=w555, lower limit=0.0) -> (In Range?=w585:bool)  [unwired: 1 out]
            n215 = In Range and Coerce(upper limit=180.0, x=w555, lower limit=110.0) -> (In Range?=w584:bool)  [unwired: 1 out]
            n216 = Or(x=w569, y=w568) -> (x .or. y?=w556:bool)
            n217 = Or(x=w563, y=w562) -> (x .or. y?=w557:bool)
            n218 = Or(x=w582, y=w581) -> (x .or. y?=w580:bool)
            n219 = Or(x=w585, y=w584) -> (x .or. y?=w583:bool)
          }
          frame "Right_LR" {
            n220 = In Range and Coerce(upper limit=227.0, x=w587, lower limit=187.0) -> (In Range?=w618:bool)  [unwired: 1 out]
            n221 = In Range and Coerce(upper limit=0.0, x=w587, lower limit=0.0) -> (In Range?=w601:bool)  [unwired: 1 out]
            n222 = In Range and Coerce(upper limit=110.0, x=w587, lower limit=30.0) -> (In Range?=w600:bool)  [unwired: 1 out]
            n223 = In Range and Coerce(upper limit=187.0, x=w587, lower limit=110.0) -> (In Range?=w595:bool)  [unwired: 1 out]
            n224 = In Range and Coerce(upper limit=300.0, x=w587, lower limit=227.0) -> (In Range?=w594:bool)  [unwired: 1 out]
            n225 = In Range and Coerce(upper limit=110.0, x=w587, lower limit=90.0) -> (In Range?=w614:bool)  [unwired: 1 out]
            n226 = In Range and Coerce(upper limit=227.0 ("x"), x=w587, lower limit=207.0) -> (In Range?=w613:bool)  [unwired: 1 out]
            n227 = In Range and Coerce(upper limit=0.0, x=w587, lower limit=0.0) -> (In Range?=w617:bool)  [unwired: 1 out]
            n228 = In Range and Coerce(upper limit=187.0, x=w587, lower limit=110.0) -> (In Range?=w616:bool)  [unwired: 1 out]
            n229 = Or(x=w601, y=w600) -> (x .or. y?=w588:bool)
            n230 = Or(x=w595, y=w594) -> (x .or. y?=w589:bool)
            n231 = Or(x=w614, y=w613) -> (x .or. y?=w612:bool)
            n232 = Or(x=w617, y=w616) -> (x .or. y?=w615:bool)
          }
          frame "Right_RL" {
            n233 = In Range and Coerce(upper limit=222.0, x=w619, lower limit=182.0) -> (In Range?=w650:bool)  [unwired: 1 out]
            n234 = In Range and Coerce(upper limit=0.0, x=w619, lower limit=0.0) -> (In Range?=w633:bool)  [unwired: 1 out]
            n235 = In Range and Coerce(upper limit=142.0, x=w619, lower limit=62.0) -> (In Range?=w632:bool)  [unwired: 1 out]
            n236 = In Range and Coerce(upper limit=300.0, x=w619, lower limit=222.0) -> (In Range?=w627:bool)  [unwired: 1 out]
            n237 = In Range and Coerce(upper limit=182.0, x=w619, lower limit=142.0) -> (In Range?=w626:bool)  [unwired: 1 out]
            n238 = In Range and Coerce(upper limit=142.0, x=w619, lower limit=122.0) -> (In Range?=w646:bool)  [unwired: 1 out]
            n239 = In Range and Coerce(upper limit=222.0 ("x"), x=w619, lower limit=202.0) -> (In Range?=w645:bool)  [unwired: 1 out]
            n240 = In Range and Coerce(upper limit=0.0, x=w619, lower limit=0.0) -> (In Range?=w649:bool)  [unwired: 1 out]
            n241 = In Range and Coerce(upper limit=182.0, x=w619, lower limit=142.0) -> (In Range?=w648:bool)  [unwired: 1 out]
            n242 = Or(x=w633, y=w632) -> (x .or. y?=w620:bool)
            n243 = Or(x=w627, y=w626) -> (x .or. y?=w621:bool)
            n244 = Or(x=w646, y=w645) -> (x .or. y?=w644:bool)
            n245 = Or(x=w649, y=w648) -> (x .or. y?=w647:bool)
          }
          frame "RIght_LL" {
            n246 = In Range and Coerce(upper limit=228.0, x=w651, lower limit=188.0) -> (In Range?=w682:bool)  [unwired: 1 out]
            n247 = In Range and Coerce(upper limit=0.0, x=w651, lower limit=0.0) -> (In Range?=w665:bool)  [unwired: 1 out]
            n248 = In Range and Coerce(upper limit=142.0, x=w651, lower limit=62.0) -> (In Range?=w664:bool)  [unwired: 1 out]
            n249 = In Range and Coerce(upper limit=188.0, x=w651, lower limit=142.0) -> (In Range?=w659:bool)  [unwired: 1 out]
            n250 = In Range and Coerce(upper limit=228.0, x=w651, lower limit=300.0) -> (In Range?=w658:bool)  [unwired: 1 out]
            n251 = In Range and Coerce(upper limit=142.0, x=w651, lower limit=122.0) -> (In Range?=w678:bool)  [unwired: 1 out]
            n252 = In Range and Coerce(upper limit=228.0 ("x"), x=w651, lower limit=208.0) -> (In Range?=w677:bool)  [unwired: 1 out]
            n253 = In Range and Coerce(upper limit=0.0, x=w651, lower limit=0.0) -> (In Range?=w681:bool)  [unwired: 1 out]
            n254 = In Range and Coerce(upper limit=188.0, x=w651, lower limit=142.0) -> (In Range?=w680:bool)  [unwired: 1 out]
            n255 = Or(x=w665, y=w664) -> (x .or. y?=w652:bool)
            n256 = Or(x=w659, y=w658) -> (x .or. y?=w653:bool)
            n257 = Or(x=w678, y=w677) -> (x .or. y?=w676:bool)
            n258 = Or(x=w681, y=w680) -> (x .or. y?=w679:bool)
          }
          frame "Right_XR" {
            n259 = In Range and Coerce(upper limit=0.0, x=w683, lower limit=0.0) -> (In Range?=w714:bool)  [unwired: 1 out]
            n260 = In Range and Coerce(upper limit=300.0, x=w683, lower limit=150.0) -> (In Range?=w697:bool)  [unwired: 1 out]
            n261 = In Range and Coerce(upper limit=97.0, x=w683, lower limit=0.0) -> (In Range?=w696:bool)  [unwired: 1 out]
            n262 = In Range and Coerce(upper limit=140.0, x=w683, lower limit=97.0) -> (In Range?=w691:bool)  [unwired: 1 out]
            n263 = In Range and Coerce(upper limit=0.0, x=w683, lower limit=0.0) -> (In Range?=w690:bool)  [unwired: 1 out]
            n264 = In Range and Coerce(upper limit=96.0, x=w683, lower limit=92.0) -> (In Range?=w710:bool)  [unwired: 1 out]
            n265 = In Range and Coerce(upper limit=0.0 ("x"), x=w683, lower limit=0.0) -> (In Range?=w709:bool)  [unwired: 1 out]
            n266 = In Range and Coerce(upper limit=0.0, x=w683, lower limit=0.0) -> (In Range?=w713:bool)  [unwired: 1 out]
            n267 = In Range and Coerce(upper limit=0.0, x=w683, lower limit=0.0) -> (In Range?=w712:bool)  [unwired: 1 out]
            n268 = Or(x=w697, y=w696) -> (x .or. y?=w684:bool)
            n269 = Or(x=w691, y=w690) -> (x .or. y?=w685:bool)
            n270 = Or(x=w710, y=w709) -> (x .or. y?=w708:bool)
            n271 = Or(x=w713, y=w712) -> (x .or. y?=w711:bool)
          }
          frame "Right_XL" {
            n272 = In Range and Coerce(upper limit=0.0, x=w715, lower limit=0.0) -> (In Range?=w746:bool)  [unwired: 1 out]
            n273 = In Range and Coerce(upper limit=230.0, x=w715, lower limit=140.0) -> (In Range?=w729:bool)  [unwired: 1 out]
            n274 = In Range and Coerce(upper limit=0.0, x=w715, lower limit=0.0) -> (In Range?=w728:bool)  [unwired: 1 out]
            n275 = In Range and Coerce(upper limit=300.0, x=w715, lower limit=230.0) -> (In Range?=w723:bool)  [unwired: 1 out]
            n276 = In Range and Coerce(upper limit=0.0, x=w715, lower limit=0.0) -> (In Range?=w722:bool)  [unwired: 1 out]
            n277 = In Range and Coerce(upper limit=230.0, x=w715, lower limit=210.0) -> (In Range?=w742:bool)  [unwired: 1 out]
            n278 = In Range and Coerce(upper limit=0.0 ("x"), x=w715, lower limit=0.0) -> (In Range?=w741:bool)  [unwired: 1 out]
            n279 = In Range and Coerce(upper limit=0.0, x=w715, lower limit=0.0) -> (In Range?=w745:bool)  [unwired: 1 out]
            n280 = In Range and Coerce(upper limit=0.0, x=w715, lower limit=0.0) -> (In Range?=w744:bool)  [unwired: 1 out]
            n281 = Or(x=w729, y=w728) -> (x .or. y?=w716:bool)
            n282 = Or(x=w723, y=w722) -> (x .or. y?=w717:bool)
            n283 = Or(x=w742, y=w741) -> (x .or. y?=w740:bool)
            n284 = Or(x=w745, y=w744) -> (x .or. y?=w743:bool)
          }
          frame "Left_XR" {
            n285 = In Range and Coerce(upper limit=0.0, x=w747, lower limit=0.0) -> (In Range?=w778:bool)  [unwired: 1 out]
            n286 = In Range and Coerce(upper limit=230.0, x=w747, lower limit=140.0) -> (In Range?=w761:bool)  [unwired: 1 out]
            n287 = In Range and Coerce(upper limit=0.0, x=w747, lower limit=0.0) -> (In Range?=w760:bool)  [unwired: 1 out]
            n288 = In Range and Coerce(upper limit=300.0, x=w747, lower limit=230.0) -> (In Range?=w755:bool)  [unwired: 1 out]
            n289 = In Range and Coerce(upper limit=0.0, x=w747, lower limit=0.0) -> (In Range?=w754:bool)  [unwired: 1 out]
            n290 = In Range and Coerce(upper limit=230.0, x=w747, lower limit=210.0) -> (In Range?=w774:bool)  [unwired: 1 out]
            n291 = In Range and Coerce(upper limit=0.0 ("x"), x=w747, lower limit=0.0) -> (In Range?=w773:bool)  [unwired: 1 out]
            n292 = In Range and Coerce(upper limit=0.0, x=w747, lower limit=0.0) -> (In Range?=w777:bool)  [unwired: 1 out]
            n293 = In Range and Coerce(upper limit=0.0, x=w747, lower limit=0.0) -> (In Range?=w776:bool)  [unwired: 1 out]
            n294 = Or(x=w761, y=w760) -> (x .or. y?=w748:bool)
            n295 = Or(x=w755, y=w754) -> (x .or. y?=w749:bool)
            n296 = Or(x=w774, y=w773) -> (x .or. y?=w772:bool)
            n297 = Or(x=w777, y=w776) -> (x .or. y?=w775:bool)
          }
          frame "Left_XL" {
            n298 = In Range and Coerce(upper limit=0.0, x=w779, lower limit=0.0) -> (In Range?=w810:bool)  [unwired: 1 out]
            n299 = In Range and Coerce(upper limit=300.0, x=w779, lower limit=150.0) -> (In Range?=w793:bool)  [unwired: 1 out]
            n300 = In Range and Coerce(upper limit=97.0, x=w779, lower limit=0.0) -> (In Range?=w792:bool)  [unwired: 1 out]
            n301 = In Range and Coerce(upper limit=140.0, x=w779, lower limit=97.0) -> (In Range?=w787:bool)  [unwired: 1 out]
            n302 = In Range and Coerce(upper limit=0.0, x=w779, lower limit=0.0) -> (In Range?=w786:bool)  [unwired: 1 out]
            n303 = In Range and Coerce(upper limit=96.0, x=w779, lower limit=92.0) -> (In Range?=w806:bool)  [unwired: 1 out]
            n304 = In Range and Coerce(upper limit=0.0 ("x"), x=w779, lower limit=0.0) -> (In Range?=w805:bool)  [unwired: 1 out]
            n305 = In Range and Coerce(upper limit=0.0, x=w779, lower limit=0.0) -> (In Range?=w809:bool)  [unwired: 1 out]
            n306 = In Range and Coerce(upper limit=150.0, x=w779, lower limit=97.0) -> (In Range?=w808:bool)  [unwired: 1 out]
            n307 = Or(x=w793, y=w792) -> (x .or. y?=w780:bool)
            n308 = Or(x=w787, y=w786) -> (x .or. y?=w781:bool)
            n309 = Or(x=w806, y=w805) -> (x .or. y?=w804:bool)
            n310 = Or(x=w809, y=w808) -> (x .or. y?=w807:bool)
          }
        }
        n311 = Wait (ms)(milliseconds to wait=u32 50) -> ()  [unwired: 1 out]
        n312 = Or(x=w157, y=w145) -> (x .or. y?=w159:bool)
        n313 = Select(t=enum16{"Scale", "Switch", "Intake", "Reserve"}."Switch", s=w152, f=enum16{"Scale", "Switch", "Intake", "Reserve"}."Reserve") -> (s? t:f=w151:enum16{"Scale", "Switch", "Intake", "Reserve"})
        n314 = call "Is Value Changed.vim"("value"=w159) -> ()  [unwired: 1 out]
        n315 = Select(t=enum16{"Scale", "Switch", "Intake", "Reserve"}."Scale", s=w150, f=w151) -> (s? t:f=w146:enum16{"Scale", "Switch", "Intake", "Reserve"})
        n316 = Select(t=enum16{"Scale", "Switch", "Intake", "Reserve"}."Intake", s=w149, f=w146) -> (s? t:f=w144:enum16{"Scale", "Switch", "Intake", "Reserve"})
        n317 = case shown="\"Reserve\", Default" w144 {
          frame "Scale" {
          }
          frame "Switch" {
          }
          frame "Intake" {
          }
          frame "Reserve", Default {
          }
        }
      }
    }
  }
